vi "esp301 set relative move.vi"(7 "Seperator in":string, 8 "error in (no error)":errorcluster, 9 "Command":string, 10 "Arg":string, 11 "ESP301 in":refnum<class "ESP301.lvclass">) -> (0 "error out":errorcluster, 2 "new commands":string, 3 "ESP301 out":refnum<class "ESP301.lvclass">)   [LabVIEW 2020, in "ESP301.lvclass"]
uses:
  ESP301.lvclass
  shared/OnOffTypeDef.ctl
  ESP301.lvclass/ESP301.ctl
  activeflag.ctl
  shared/CompressAndUpdate(Poly)/CompressAndUpdate(Enum).vi
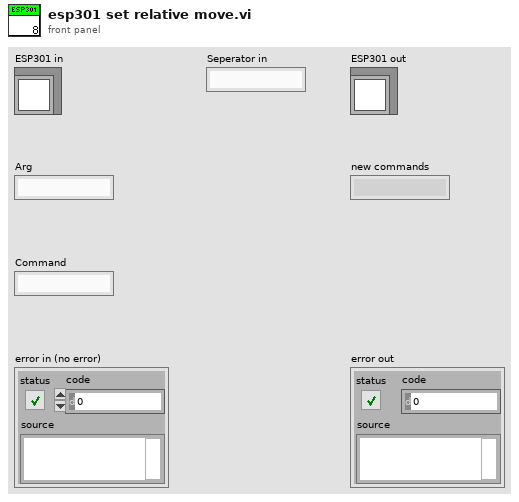
[diagram p1: front panel]
types:
  T1 = typedef "OnOffTypeDef.ctl" = enum16{"off", "on"}
  T2 = typedef "activeflag.ctl" = enum16{"on", "off", "n/a"}
  T3 = typedef "ESP301.lvclass/SettingsTypdef.ctl" = cluster{"devport":string, "Position":cluster{"Axis 1":cluster{"Value":dbl, "Min":dbl, "Max":dbl, "StepSize":dbl, "Tolerance":dbl, "ValueActual":dbl}, "Axis 2":cluster{"Value":dbl, "Min":dbl, "Max":dbl, "StepSize":dbl, "Tolerance":dbl, "ValueActual":dbl}, "Axis 3":cluster{"Value":dbl, "Min":dbl, "Max":dbl, "StepSize":dbl, "Tolerance":dbl, "ValueActual":dbl}}, "Power":cluster{"Axis 1":T1, "Axis 2":T1, "Axis 3":T1}, "Status":cluster{"Axis 1":T4, "Axis 2":T4, "Axis 3":T4}, "Backlash":cluster{"Axis 1":cluster{"Value":dbl, "Min":dbl, "Max":dbl, "StepSize":dbl, "Tolerance":dbl, "ValueActual":dbl}, "Axis 2":cluster{"Value":dbl, "Min":dbl, "Max":dbl, "StepSize":dbl, "Tolerance":dbl, "ValueActual":dbl}, "Axis 3":cluster{"Value":dbl, "Min":dbl, "Max":dbl, "StepSize":dbl, "Tolerance":dbl, "ValueActual":dbl}}, "Home":cluster{"Axis 1":cluster{"Value":dbl, "Min":dbl, "Max":dbl, "StepSize":dbl, "Tolerance":dbl, "ValueActual":dbl}, "Axis 2":cluster{"Value":dbl, "Min":dbl, "Max":dbl, "StepSize":dbl, "Tolerance":dbl, "ValueActual":dbl}, "Axis 3":cluster{"Value":dbl, "Min":dbl, "Max":dbl, "StepSize":dbl, "Tolerance":dbl, "ValueActual":dbl}}, "MoveToHardLimit":cluster{"Axis 1":T5, "Axis 2":T5, "Axis 3":T5}, "relativeMove":cluster{"Axis 1neg":T1, "Axis 2neg":T1, "Axis 3neg":T1, "Axis 1pos":T1, "Axis 2pos":T1, "Axis 3pos":T1}, "stepsize":cluster{"Value":dbl, "Min":dbl, "Max":dbl, "StepSize":dbl, "Tolerance":dbl, "ValueActual":dbl}, "automotoroff":T1, "ResetBeforeMove":T1, "Enable":cluster{"Axis 1":T1, "Axis 2":T1, "Axis 3":T1}, "InitWithDBValues":T1}
  T4 = typedef "status_TypDef.ctl" = enum16{"Not referenced", "Homing", "Moving", "Ready"}
  T5 = typedef "Hardware limit.ctl" = enum16{"pos", "neg"}
  T6 = cluster{"Axis 1":cluster{"Value":dbl, "Min":dbl, "Max":dbl, "StepSize":dbl, "Tolerance":dbl, "ValueActual":dbl}, "Axis 2":cluster{"Value":dbl, "Min":dbl, "Max":dbl, "StepSize":dbl, "Tolerance":dbl, "ValueActual":dbl}, "Axis 3":cluster{"Value":dbl, "Min":dbl, "Max":dbl, "StepSize":dbl, "Tolerance":dbl, "ValueActual":dbl}}
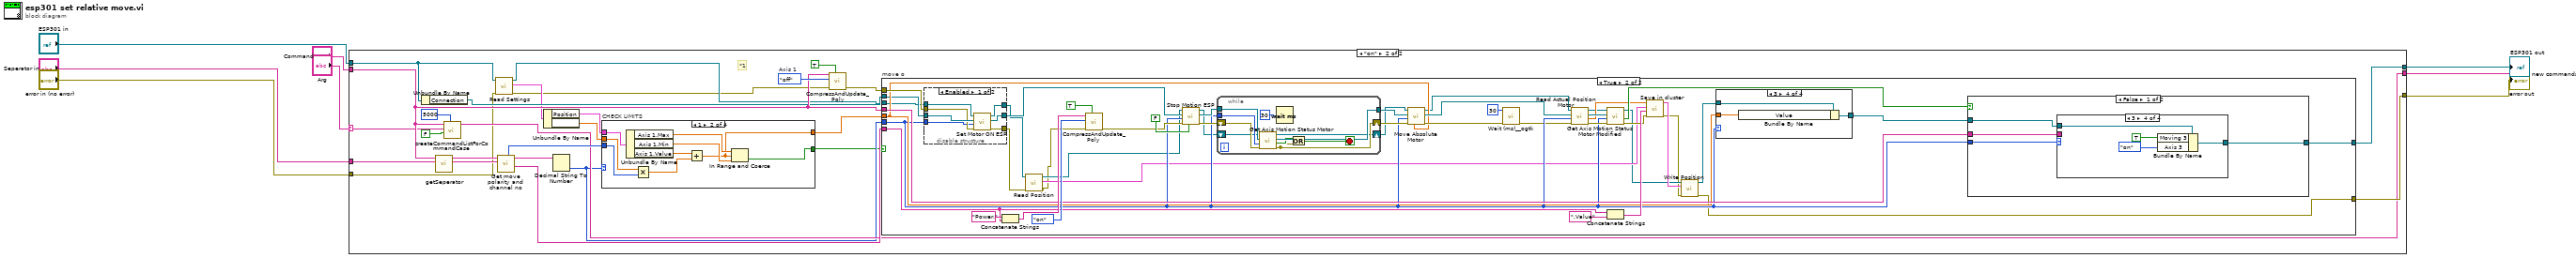
[diagram p0: block diagram]
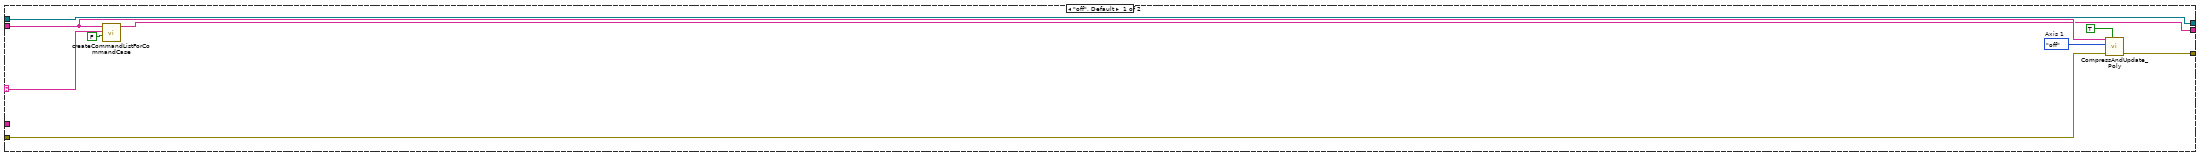
[diagram p2: hidden frame]
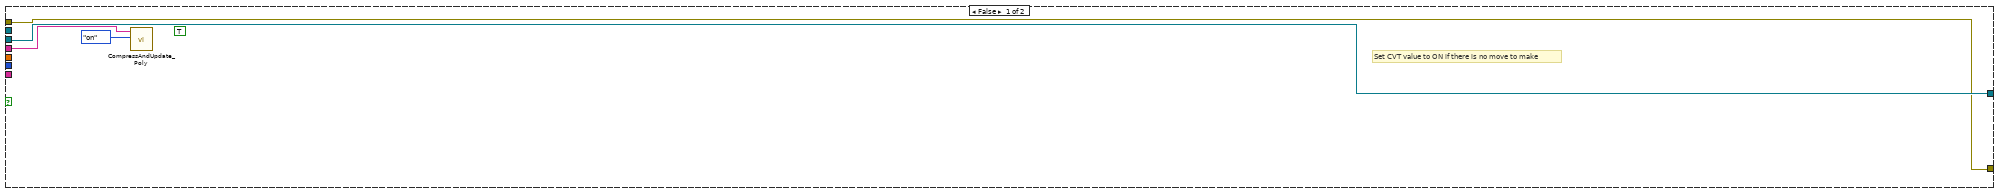
[diagram p3: hidden frame]
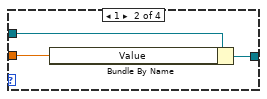
[diagram p5: hidden frame]
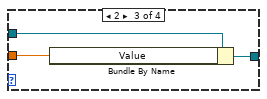
[diagram p6: hidden frame]
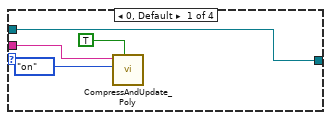
[diagram p8: hidden frame]
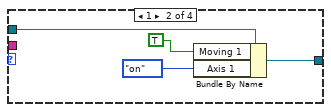
[diagram p9: hidden frame]
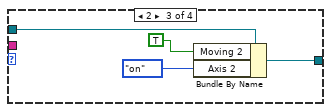
[diagram p10: hidden frame]
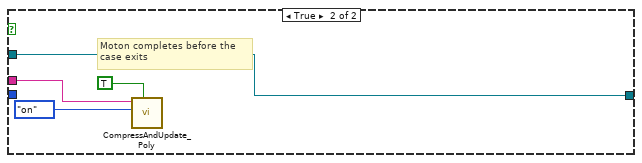
[diagram p11: hidden frame]
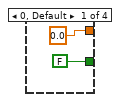
[diagram p12: hidden frame]
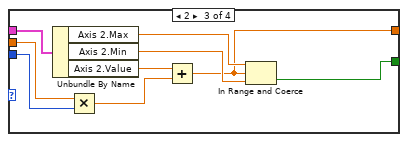
[diagram p13: hidden frame]
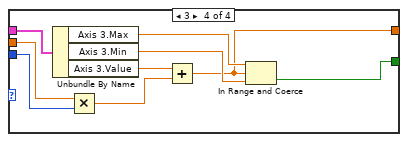
[diagram p14: hidden frame]
diagram:
  n1 = case shown="\"on\"" "Arg" {
    selector: "Arg" -> [w9 w28]
    tunnel: [w10 w29] -> w1
    tunnel: [w13 w40] -> w2
    tunnel: "Seperator in" -> [_ w44]
    tunnel: [w17 w35] -> w4
    tunnel: "Command" -> [w11 w30]
    tunnel: "ESP301 in" -> [w17 w21]
    tunnel: "error in (no error)" -> [w14 w18]
    frame "off", Default {
      w15 = OnOffTypeDef."off"  # Axis 1
      n2 = call "createCommandListForCommandCase.vi"("immediate Check (only once)"=FALSE, "setvalue"=w9, "command"=w11) -> ("new commands"=w10:string)  [unwired: 8 in]
      n3 = call-poly "CompressAndUpdate_Poly.vi"("force CVT update (false)"=TRUE ("force CVT update"), "error in"=w14, "enum variant"=w15, "command or variable name"=w11) -> ("error out"=w13:errorcluster)  [unwired: 7 in]
    }
    frame "on" {
      w41 = OnOffTypeDef."off"  # Axis 1
      # "*1"
      n4 = Unbundle By Name(w21) -> ("Connection"=w24:refnum<visa-resource-name>)
      n5 = call "getSeperator.vi"("Channel Seperator (\"\")"=w44, "Command"=w30) -> ("Channel"=w31:string, "Seperator (e.g. \"Channel1\")"=w32:string)  [unwired: 8 in]
      n6 = call "createCommandListForCommandCase.vi"("timeout (optional)"=5000, "immediate Check (only once)"=FALSE, "setvalue"=w28, "command"=w30) -> ("new commands"=w29:string)  [unwired: 7 in]
      n7 = call-dynamic "Read Settings.vi"("error in (no error)"=w18, "ESP301 in"=w21) -> ("error out"=w19:errorcluster, "Settings"=w20:T3, "ESP301 out"=w22:refnum<class "ESP301.lvclass">)  [unwired: 7 in]
      n8 = call "Get move polarity and channel no.vi"("Channel in"=w31, "Channel string In"=w32) -> ("Channel Out"=w36:string, "Channel out"=w39:string, "Numeric"=w33:i32)  [unwired: 7 in]
      n9 = Unbundle By Name(w20) -> ("Position"=w38:T6, "stepsize.Value"=w37:dbl)
      n10 = Decimal String To Number(string=w39) -> (number=w26:i32)  [unwired: 2 in, 1 out]
      n11 = case "CHECK LIMITS" shown="1" w26 {
        tunnel: w38 -> [_ w157 w166 w175]
        tunnel: w37 -> [_ w155 w164 w173]
        tunnel: w33 -> [_ w156 w165 w174]
        tunnel: [0.0 w150 w159 w168] -> w34
        tunnel: [FALSE w149 w158 w167] -> w23
        frame 0, Default {
        }
        frame 1 {
          n12 = Unbundle By Name(w157) -> ("Axis 1.Max"=w152:dbl, "Axis 1.Min"=w151:dbl, "Axis 1.Value"=w154:dbl)
          n13 = Multiply(x=w155, y=w156) -> (x*y=w153:dbl)
          n14 = Add(x=w154, y=w153) -> (x+y=w150:dbl)
          n15 = In Range and Coerce(upper limit=w152, x=w150, lower limit=w151) -> (In Range?=w149:bool)  [unwired: 1 out]
        }
        frame 2 {
          n16 = Unbundle By Name(w166) -> ("Axis 2.Max"=w160:dbl, "Axis 2.Min"=w161:dbl, "Axis 2.Value"=w163:dbl)
          n17 = Multiply(x=w164, y=w165) -> (x*y=w162:dbl)
          n18 = Add(x=w163, y=w162) -> (x+y=w159:dbl)
          n19 = In Range and Coerce(upper limit=w160, x=w159, lower limit=w161) -> (In Range?=w158:bool)  [unwired: 1 out]
        }
        frame 3 {
          n20 = Unbundle By Name(w175) -> ("Axis 3.Max"=w170:dbl, "Axis 3.Min"=w169:dbl, "Axis 3.Value"=w172:dbl)
          n21 = Multiply(x=w173, y=w174) -> (x*y=w171:dbl)
          n22 = Add(x=w172, y=w171) -> (x+y=w168:dbl)
          n23 = In Range and Coerce(upper limit=w170, x=w168, lower limit=w169) -> (In Range?=w167:bool)  [unwired: 1 out]
        }
      }
      n24 = call-poly "CompressAndUpdate_Poly.vi"("force CVT update (false)"=TRUE ("force CVT update"), "error in"=w19, "enum variant"=w41, "command or variable name"=w30) -> ("error out"=w25:errorcluster)  [unwired: 7 in]
      n25 = case "move o" shown="True" w23 {
        tunnel: w25 -> [w47 w74]
        tunnel: [w47 w51] -> w40
        tunnel: w22 -> [w48 w65]
        tunnel: w26 -> [_ w67]
        tunnel: w34 -> [_ w68]
        tunnel: w36 -> [_ w72]
        tunnel: [w48 w71] -> w35
        tunnel: w30 -> [w45 w70]
        tunnel: w24 -> [_ w66]
        frame False {
          (unwired) TRUE ("force CVT update")
          # "Set CVT value to ON if there is no move to make"
          n26 = call-poly "CompressAndUpdate_Poly.vi"("enum variant"=OnOffTypeDef."on" ("Axis 1"), "command or variable name"=w45) -> ()  [unwired: 9 in, 1 out]
        }
        frame True {
          n27 = disable-structure shown="Enabled" {
            disable-tunnel: w66 -> [w110 w112]
            disable-tunnel: [w109 w112] -> w79
            disable-tunnel: w74 -> [w108 w111]
            disable-tunnel: [w107 w111] -> w57
            disable-tunnel: w67 -> [w106 _]
            disable-tunnel: w65 -> [w105 _]
            disable-tunnel: [w104 _] -> w58
            frame Enabled {
              n28 = call-dynamic "Set Motor ON ESP.vi"("error in (no error)"=w108, "Axis (1)"=w106, "VISA resource name"=w110, "ESP301 in"=w105) -> ("error out"=w107:errorcluster, "VISA resource name out"=w109:refnum<visa-resource-name>, "ESP301 out"=w104:refnum<class "ESP301.lvclass">)  [unwired: 5 in]
            }
            frame Disabled {
            }
          }
          n29 = Concatenate Strings("Power." ("string"), w72) -> (w76:string)
          n30 = call "Read Position.vi"("error in (no error)"=w57, "ESP301 in"=w58) -> ("error out"=w49:errorcluster, "Position"=w56:T6, "ESP301 out"=w50:refnum<class "ESP301.lvclass">)  [unwired: 7 in]
          n31 = call-poly "CompressAndUpdate_Poly.vi"("force CVT update (false)"=TRUE ("force CVT update"), "error in"=w49, "enum variant"=OnOffTypeDef."on" ("Axis 1"), "command or variable name"=w76) -> ("error out"=w73:errorcluster)  [unwired: 7 in]
          n32 = call-dynamic "Stop Motion ESP.vi"("Stop all axes (F)"=FALSE, "error in (no error)"=w73, "Axis (1)"=w67, "VISA resource name"=w79, "ESP301 in"=w50) -> ("error out"=w90:errorcluster, "VISA resource name out"=w88:refnum<visa-resource-name>, "ESP301 out"=w64:refnum<class "ESP301.lvclass">)  [unwired: 4 in]
          n33 = while {
            tunnel: w88 -> [w146]
            tunnel: w67 -> [w145]
            tunnel: [w143] -> w87
            shift-right: [w141] -> w89
            shift-left: w90 -> [w144]
            shift-right: [w137] -> w63
            shift-left: w64 -> [w138]
            stop <- w140 stop-if-true
            n34 = call-dynamic "Get Axis Motion Status Motor.vi"("error in (no error)"=w144, "Axis (1)"=w145, "VISA resource name"=w146, "ESP301 in"=w138) -> ("error out"=w141:errorcluster, "Motion Done"=w142:bool, "VISA resource name out"=w143:refnum<visa-resource-name>, "ESP301 out"=w137:refnum<class "ESP301.lvclass">)  [unwired: 4 in]
            n35 = Wait (ms)(milliseconds to wait=u32 30) -> ()  [unwired: 1 out]
            n36 = Or(x=w142, y=w141) -> (x .or. y?=w140:bool)
          }
          n37 = call-dynamic "Move Absolute Motor.vi"("Position (0 units)"=w68, "error in (no error)"=w89, "Axis (1)"=w67, "VISA resource name"=w87, "ESP301 in"=w63) -> ("error out"=w84:errorcluster, "VISA resource name out"=w85:refnum<visa-resource-name>, "ESP301 out"=w62:refnum<class "ESP301.lvclass">)  [unwired: 4 in]
          n38 = call <userlib>:"Wait (ms)__ogtk.vi"("error in (no error)"=w84, "milliseconds to wait"=u32 30) -> ("error out"=w61:errorcluster)  [unwired: 8 in, 1 out]
          n39 = call-dynamic "Read Actual Position Motor.vi"("error in (no error)"=w61, "Axis (1)"=w67, "VISA resource name"=w85, "ESP301 in"=w62) -> ("error out"=w83:errorcluster, "Position (units)"=w81:dbl, "VISA resource name out"=w86:refnum<visa-resource-name>, "ESP301 out"=w59:refnum<class "ESP301.lvclass">)  [unwired: 4 in]
          n40 = call-dynamic "Get Axis Motion Status Motor Modified.vi"("error in (no error)"=w83, "Axis (1)"=w67, "VISA resource name"=w86, "ESP301 in"=w59) -> ("error out"=w80:errorcluster, "Motion Done"=w82:bool, "ESP301 out"=w54:refnum<class "ESP301.lvclass">)  [unwired: 4 in, 1 out]
          n41 = Concatenate Strings(w72, ".Value" ("string")) -> (w92:string)
          n42 = call "Save in cluster.vi"("error in (no error)"=w80, "String"=w92, "Home in"=w56, "Numeric"=w81) -> ("error out"=w52:errorcluster, "Home out"=w55:T6)  [unwired: 6 in]
          n43 = call "Write Position.vi"("error in (no error)"=w52, "Position"=w55, "ESP301 in"=w54) -> ("error out"=w51:errorcluster, "ESP301 out"=w53:refnum<class "ESP301.lvclass">)  [unwired: 7 in]
          n44 = case shown="3" w67 {
            tunnel: w53 -> [w94 w97 w100 w103]
            tunnel: [w94 w96 w99 w102] -> w69
            tunnel: w68 -> [_ w95 w98 w101]
            frame 0, Default {
            }
            frame 1 {
              n45 = Bundle By Name(cluster=w97, "Value"=w95) -> (w96:refnum<class "ESP301.lvclass">)
            }
            frame 2 {
              n46 = Bundle By Name(cluster=w100, "Value"=w98) -> (w99:refnum<class "ESP301.lvclass">)
            }
            frame 3 {
              n47 = Bundle By Name(cluster=w103, "Value"=w101) -> (w102:refnum<class "ESP301.lvclass">)
            }
          }
          n48 = case shown="False" w82 {
            tunnel: w67 -> [w116 _]
            tunnel: w69 -> [w115 w133]
            tunnel: [w114 w133] -> w71
            tunnel: w70 -> [w113 w135]
            frame False {
              n49 = case shown="3" w116 {
                tunnel: w115 -> [w117 w124 w128 w132]
                tunnel: [w117 w123 w127 w131] -> w114
                tunnel: w113 -> [w118 _ _ _]
                frame 0, Default {
                  n50 = call-poly "CompressAndUpdate_Poly.vi"("force CVT update (false)"=TRUE ("force CVT update"), "enum variant"=OnOffTypeDef."on" ("Axis 1"), "command or variable name"=w118) -> ()  [unwired: 8 in, 1 out]
                }
                frame 1 {
                  n51 = Bundle By Name(cluster=w124, "Moving 1"=TRUE, "Axis 1"=activeflag."on" ("ActiveFlag")) -> (w123:refnum<class "ESP301.lvclass">)
                }
                frame 2 {
                  n52 = Bundle By Name(cluster=w128, "Moving 2"=TRUE, "Axis 2"=activeflag."on" ("ActiveFlag")) -> (w127:refnum<class "ESP301.lvclass">)
                }
                frame 3 {
                  n53 = Bundle By Name(cluster=w132, "Moving 3"=TRUE, "Axis 3"=activeflag."on" ("ActiveFlag")) -> (w131:refnum<class "ESP301.lvclass">)
                }
              }
            }
            frame True {
              # "Moton completes before the\ncase exits"
              n54 = call-poly "CompressAndUpdate_Poly.vi"("force CVT update (false)"=TRUE ("force CVT update"), "enum variant"=OnOffTypeDef."on" ("Axis 1"), "command or variable name"=w135) -> ()  [unwired: 8 in, 1 out]
            }
          }
        }
      }
    }
  }
  "ESP301 out" <- w4
  "error out" <- w2
  "new commands" <- w1
